vi "Test auto state machine.vi"() -> ()   [LabVIEW 2017]
panel:
  in  "Cluster":T1
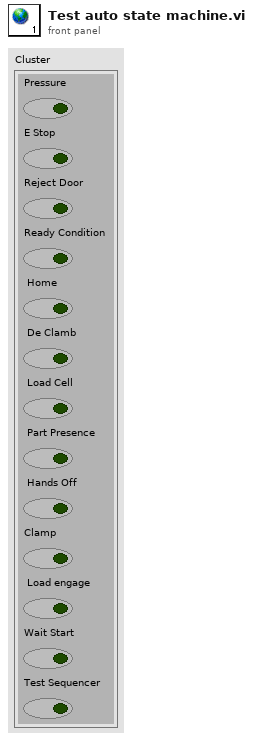
[diagram p1: front panel]
types:
  T1 = cluster{"Pressure":bool, "E Stop":bool, "Reject Door":bool, "Ready Condition":bool, " Home":bool, " De Clamb":bool, " Load Cell":bool, " Part Presence":bool, " Hands Off":bool, "Clamp":bool, " Load engage":bool, "Wait Start":bool, "Test Sequencer":bool}
diagram:
